vi "Fetch Multi Eval Meas List SEM Margin Area Results.vi"(6 "Area (1)":T1=1, 7 "Offset Frequency (Positive)":i32(ring)=1 items=["Negative", "Positive"], 8 "error in (no error)":errorcluster, 9 "Result Type (Current)":i32(ring) items=["Current"=0, "Average"=1, "Minimum"=5], 10 "Instance (1)":T2=1, 11 "VISA resource name":refnum<visa-resource-name>) -> (0 "error out":errorcluster, 1 "Results":cluster{"Margin X":dbl, "Margin Y":dbl}[](array[cluster]) {"Margin Y" format="%#_6e"; "Margin X" format="%#_6e"}, 2 "Reliability":i32, 3 "VISA resource name out":refnum<visa-resource-name>)   [LabVIEW 2020, in "Rohde&Schwarz CMWXP NR FR1 Measurement.lvlib"]
doc: "Return spectrum emission mask margin positions for all measured list mode segments.\n\nThe results for the current, average and maximum traces (resulting in minimum margins) for negative and positive offset frequencies can be returned.\n\nAttributes:\nRSCMWXPNRFR1M_ATTR_FETCH_MULTI_EVAL_MEAS_LIST_SEM_MARGIN_AREA_POSITIVE_CURRENT_RESULTS\nRSCMWXPNRFR1M_ATTR_FETCH_MULTI_EVAL_MEAS_LIST_SEM_MARGIN_AREA_POSITIVE_AVERAGE_RESULTS\nRSCMWXPNRFR1M_ATTR_FETCH_MULTI_EVAL_MEAS_LIST_SEM_MARGIN_AREA_POSITIVE_MINIMUM_RESULTS\nRSCMWXPNRFR1M_ATTR_FETCH_MULTI_EVAL_MEAS_LIST_SEM_MARGIN_AREA_NEGATIVE_CURRENT_RESULTS\nRSCMWXPNRFR1M_ATTR_FETCH_MULTI_EVAL_MEAS_LIST_SEM_MARGIN_AREA_NEGATIVE_AVERAGE_RESULTS\nRSCMWXPNRFR1M_ATTR_FETCH_MULTI_EVAL_MEAS_LIST_SEM_MARGIN_AREA_NEGATIVE_MINIMUM_RESULTS\n\nRemote-control commands:\nFETCh:NRSub:MEAS<i>:MEValuation:LIST:SEMask:MARGin:AREA<no>:POSitiv:CURRent?\nFETCh:NRSub:MEAS<i>:MEValuation:LIST:SEMask:MARGin:AREA<no>:POSitiv:AVERage?\nFETCh:NRSub:MEAS<i>:MEValuation:LIST:SEMask:MARGin:AREA<no>:POSitiv:MINimum?\nFETCh:NRSub:MEAS<i>:MEValuation:LIST:SEMask:MARGin:AREA<no>:NEGativ:CURRent?\nFETCh:NRSub:MEAS<i>:MEValuation:LIST:SEMask:MARGin:AREA<no>:NEGativ:AVERage?\nFETCh:NRSub:MEAS<i>:MEValuation:LIST:SEMask:MARGin:AREA<no>:NEGativ:MINimum?"
uses:
  <instrlib>/Rohde&Schwarz CMWXP NR FR1 Measurement/Rohde&Schwarz CMWXP NR FR1 Measurement.lvlib
  <instrlib>/Rohde&Schwarz CMWXP NR FR1 Measurement/Private/_Instance.ctl
  <instrlib>/Rohde&Schwarz CMWXP NR FR1 Measurement/Private/_Area.ctl
  <instrlib>/Rohde&Schwarz CMWXP NR FR1 Measurement/Private/rsidr_core.llb/rsidr_core.lvlib
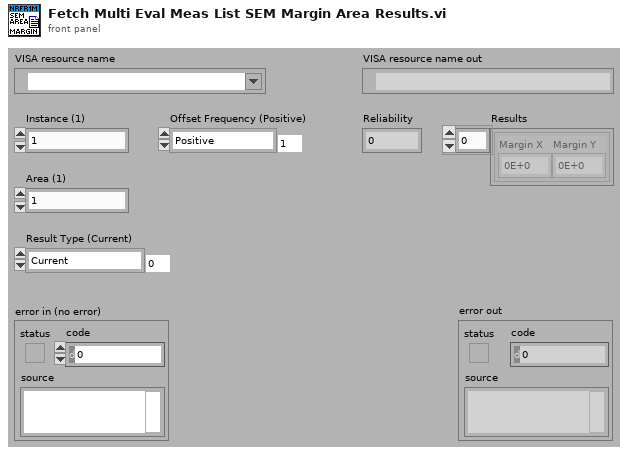
[diagram p1: front panel]
types:
  T1 = typedef "Rohde&Schwarz CMWXP NR FR1 Measurement.lvlib/_Area.ctl" = i32
  T2 = typedef "Rohde&Schwarz CMWXP NR FR1 Measurement.lvlib/_Instance.ctl" = i32
  T3 = cluster{"Margin Pos X":dbl, "Margin Pos Y":dbl}[]
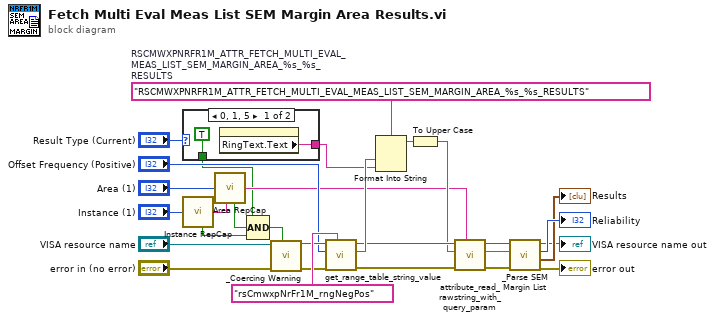
[diagram p0: block diagram]
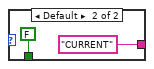
[diagram p2: hidden frame]
diagram:
  w26 = "RSCMWXPNRFR1M_ATTR_FETCH_MULTI_EVAL_MEAS_LIST_SEM_MARGIN_AREA_%s_%s_RESULTS"  # RSCMWXPNRFR1M_ATTR_FETCH_MULTI_EVAL_MEAS_LIST_SEM_MARGIN_AREA_%s_%s_RESULTS
  n1 = case shown="0, 1, 5" "Result Type (Current)" {
    tunnel: [w30 "CURRENT"] -> w24
    tunnel: [TRUE FALSE] -> w5
    frame 0, 1, 5 {
      n2 = property on="Result Type (Current)" class="Ring (strict)"() -> ("RingText.Text"=w30:string)  [unwired: 2 in, 2 out]
    }
    frame Default {
    }
  }
  n3 = call <instrlib>:"Instance RepCap.vi"("Instance In"="Instance (1)") -> ("In Range?"=w22:bool, "RepCap Identifier Out"=w10:string)  [unwired: 1 in]
  n4 = call <instrlib>:"Area RepCap.vi"("SEM Area In"="Area (1)", "RepCap String In (\"\")"=w10) -> ("In Range?"=w9:bool, "RepCap Identifier Out"=w7:string)
  n5 = Compound Arithmetic op=AND(w5, w9, w22) -> (w23:bool)
  n6 = call <instrlib>:"_Coercing Warning.vi"("In Range?"=w23, "error in (no error)"="error in (no error)", "VISA resource name"="VISA resource name") -> ("error out"=w27:errorcluster, "VISA resource name out"=w28:refnum<visa-resource-name>)  [unwired: 7 in]
  n7 = call <instrlib>:"get_range_table_string_value.vi"("Range Table ID in"="rsCmwxpNrFr1M_rngNegPos", "error in"=w27, "I32 input"="Offset Frequency (Positive)", "VISA resource name"=w28) -> ("error out"=w18:errorcluster, "String Value out"=w25:string, "VISA resource name out"=w21:refnum<visa-resource-name>)  [unwired: 5 in]
  n8 = Format Into String(format string=w26, w25, w24) -> (resulting string=w20:string)  [unwired: 2 in, 1 out]
  n9 = To Upper Case(1:w20) -> (0:w19:string)
  n10 = call <instrlib>:"attribute_read_rawstring_with_query_param.vi"("Repeated Capability"=w7, "error in"=w18, "Attribute ID"=w19, "VISA resource name"=w21) -> ("error out"=w17:errorcluster, "Raw String out"=w16:string, "VISA resource name out"=w15:refnum<visa-resource-name>)  [unwired: 5 in]
  n11 = call <instrlib>:"_Parse SEM Margin List.vi"("error in (no error)"=w17, "Input String"=w16, "VISA resource name"=w15) -> ("error out"=→"error out":errorcluster, "Results"=→"Results":T3, "Reliability"=→"Reliability":i32, "VISA resource name out"=→"VISA resource name out":refnum<visa-resource-name>)  [unwired: 5 in]
